vi "SubVI_Izh_Model_Select_003.vi"(1 "Encoder parameters":T1) -> (0 "output cluster":cluster{dbl, dbl, dbl, dbl})   [LabVIEW 2018]
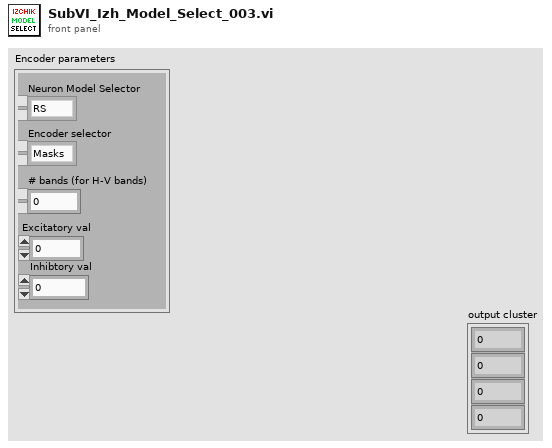
[diagram p1: front panel]
types:
  T1 = cluster{"Encoder selector":enum16{"Masks", "H-V bands", "Simple reading"}, "# bands (for H-V bands)":i32, "Excitatory val":dbl, "Inhibtory val":dbl, "Neuron Model Selector":enum16{"RS", "LTS", "RZ", "TC2", "TC1", "FS", "CH", "IB"}}
  T2 = enum16{"RS", "LTS", "RZ", "TC2", "TC1", "FS", "CH", "IB"}
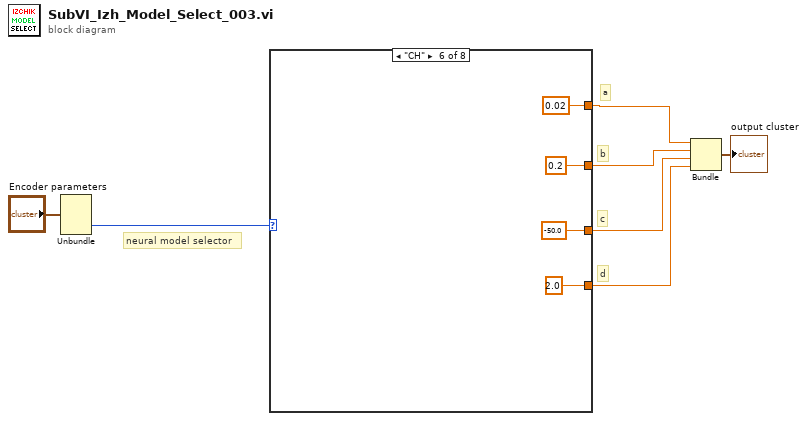
[diagram p0: block diagram]
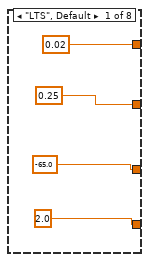
[diagram p2: hidden frame]
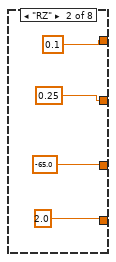
[diagram p3: hidden frame]
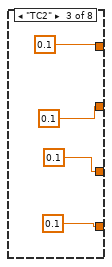
[diagram p4: hidden frame]
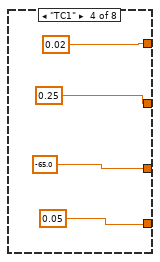
[diagram p5: hidden frame]
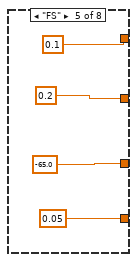
[diagram p6: hidden frame]
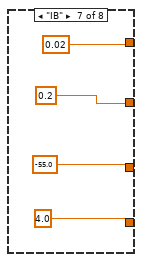
[diagram p7: hidden frame]
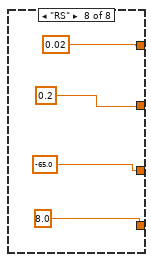
[diagram p8: hidden frame]
diagram:
  # "neural model selector"
  # "d"
  # "c"
  # "b"
  # "a"
  n1 = Unbundle("Encoder parameters") -> ("Neuron Model Selector"=w1:T2)  [unwired: 4 out]
  n2 = case shown="\"CH\"" w1 {
    tunnel: [0.02 0.1 0.1 0.02 0.1 0.02 0.02 0.02] -> w7
    tunnel: [0.25 0.25 0.1 0.25 0.2 0.2 0.2 0.2] -> w6
    tunnel: [-65.0 -65.0 0.1 -65.0 -65.0 -50.0 -55.0 -65.0] -> w5
    tunnel: [2.0 2.0 0.1 0.05 0.05 2.0 4.0 8.0] -> w4
    frame "LTS", Default {
    }
    frame "RZ" {
    }
    frame "TC2" {
    }
    frame "TC1" {
    }
    frame "FS" {
    }
    frame "CH" {
    }
    frame "IB" {
    }
    frame "RS" {
    }
  }
  n3 = Bundle(w7, w6, w5, w4) -> (→"output cluster":cluster{dbl, dbl, dbl, dbl})  [unwired: 1 in]
